vi "DBL.vi"(4 "Value":T1) -> (1 "Constant":refnum<class "Const_CPLX_SGL.lvclass">)   [LabVIEW 2021, in "Const_CPLX_SGL.lvclass"]
uses:
  Const_CPLX_SGL.lvclass
  Type.ctl
  Const_CPLX_SGL.lvclass/Const_CPLX_SGL.ctl
  Properties/Write Value.vi
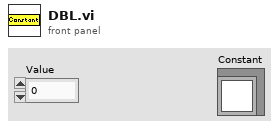
[diagram p1: front panel]
types:
  T1 = typedef "Const_CPLX_SGL.lvclass/Type.ctl" = dbl
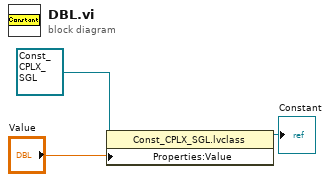
[diagram p0: block diagram]
diagram:
  n1 = property class="Const_CPLX_SGL.lvclass"(reference=refnum<class "Const_CPLX_SGL.lvclass"> refnum ("Constants.lvlib:Numeric.lvclass"), "Properties:Value"="Value") -> (reference out=→"Constant":refnum<class "Const_CPLX_SGL.lvclass">)  [unwired: 1 in, 1 out]
